vi "Day 2.2 - Win-Loose-Draw.vi"(11 "input":string[](array[string])) -> (3 "output":i16)   [LabVIEW 2021]
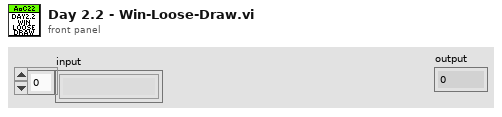
[diagram p1: front panel]
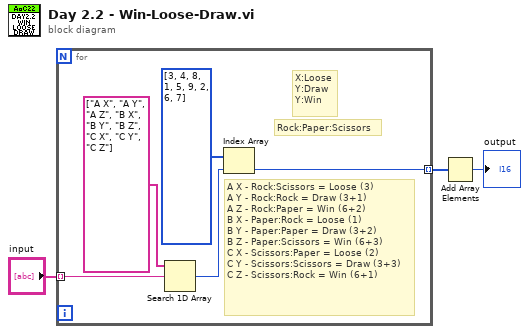
[diagram p0: block diagram]
diagram:
  n1 = for {
    tunnel: "input" -> [w8] mode=indexing
    tunnel: [w4] -> w3 mode=indexing
    # "Rock:Paper:Scissors"
    # "X:Loose\nY:Draw\nY:Win"
    # "A X - Rock:Scissors = Loose (3)\nA Y - Rock:Rock = Draw (3+1)\nA Z - Rock:Paper = Win (6+2)\nB X - Paper:Rock = Loose (1)\nB Y - Paper:Paper = Draw (3+2)\nB Z - Paper:Scissors = Win (6+3)\nC X - Scissors:Paper = Loose (2)\nC Y - Scissors:Scissors = Draw (3+3)\nC Z - Scissors:Rock = Win (6+1)"
    n2 = Search 1D Array(1D array=string[] ["A X", "A Y", "A Z", "B X", "B Y", "B Z", "C X", "C Y", "C Z"], element=w8) -> (index of element=w5:i32)  [unwired: 1 in]
    n3 = Index Array(array=i32[] [3, 4, 8, 1, 5, 9, 2, 6, 7], index=w5) -> (element=w4:i32)
  }
  n4 = Add Array Elements(numeric array=w3) -> (sum=→"output":i32)
